vi "proper demo.vi"() -> ()   [LabVIEW 2018]
uses:
  <vilib>/Instr/_visa.llb/VISA Configure Serial Port (Instr).vi
panel:
  in  "timeout (10sec)":u32=10000
  in  "stop":bool
  in  "speed 1":string="+0.234"
  in  "speed 2":string="-0.237"
  in  "speed 3":string="+1.000"
  in  "speed 4":string="+0.324"
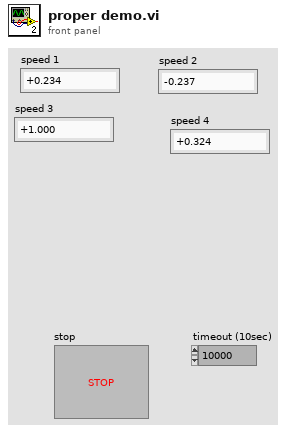
[diagram p1: front panel]
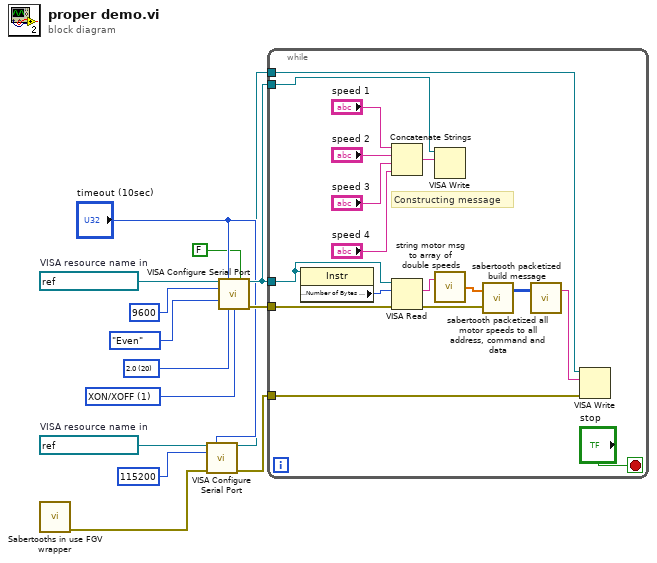
[diagram p0: block diagram]
diagram:
  w3 = u16 1 items=["None", "XON/XOFF", "RTS/CTS", "XON/XOFF & RTS/CTS", "DTR/DSR", "XON/XOFF & DTR/DSR"] ("flow control (0:none)")
  w5 = u16 20 items=["1.0"=10, "1.5"=15, "2.0"=20] ("stop bits (10: 1 bit)")
  w9 = refnum<visa-resource-name> "ASRL1::INSTR"  # VISA resource name in
  w14 = refnum<visa-resource-name> "ASRL2::INSTR"  # VISA resource name in
  n1 = call "Sabertooths in use FGV wrapper.vi"() -> ("error out"=w1:errorcluster)  [unwired: 11 in]
  n2 = call-poly "VISA Configure Serial Port"("VISA resource name"=w9, "timeout (10sec)"="timeout (10sec)", "baud rate (9600)"=u32 115200, "error in (no error)"=w1) -> ("VISA resource name out"=w7:refnum<visa-resource-name>, "error out"=w6:errorcluster)  [unwired: 10 in]
  n3 = call-poly "VISA Configure Serial Port"("VISA resource name"=w14, "timeout (10sec)"="timeout (10sec)", "Enable Termination\nChar (T)"=FALSE ("Enable Termination\nChar (T)"), "baud rate (9600)"=u32 9600, "parity (0:none)"=enum16{"None", "Odd", "Even", "Mark", "Space"}."Even", "stop bits (10: 1 bit)"=w5, "flow control (0:none)"=w3) -> ("VISA resource name out"=w12:refnum<visa-resource-name>, "error out"=w11:errorcluster)  [unwired: 7 in]
  n4 = while {
    tunnel: w12 -> [w30]
    tunnel: w12 -> [w28]
    tunnel: w11 -> [w27]
    tunnel: w7 -> [w21]
    tunnel: w6 -> [w19]
    stop <- "stop" stop-if-true
    # "Constructing message"
    n5 = property class="Instr"(reference=w30) -> ("Serial Settings:Number of Bytes at Serial Port"=w29:u32)  [unwired: 1 in, 2 out]
    n6 = Concatenate Strings("speed 1", "speed 2", "speed 3", "speed 4") -> (w26:string)
    n7 = VISA Read(VISA resource name=w30, byte count=w29, error in (no error)=w27) -> (read buffer=w18:string, error out=w15:errorcluster)  [unwired: 2 out]
    n8 = VISA Write(VISA resource name=w28, write buffer=w26) -> ()  [unwired: 1 in, 3 out]
    n9 = call "string motor msg to array of double speeds.vi"("read buffer"=w18) -> ("All speeds array (double)"=w17:dbl[])  [unwired: 1 in]
    n10 = call "sabertooth packetized all motor speeds to all address, command and data.vi"("error in (no error)"=w15, "All Motor Speeds"=w17) -> ("Data to write"=w16:u8[][][])  [unwired: 1 out]
    n11 = call "sabertooth packetized build message.vi"("Data to write"=w16) -> ("Uart Write Data"=w20:string)  [unwired: 1 in, 1 out]
    n12 = VISA Write(VISA resource name=w21, write buffer=w20, error in (no error)=w19) -> ()  [unwired: 3 out]
  }
